vi "InterpretDiagram.vi"(5 "Diagram":refnum<class "Diagram.lvclass">, 6 "error in":errorcluster, 9 "VI Interpreter in":refnum<class "VI Interpreter.lvclass">) -> (0 "error out":errorcluster, 3 "VI Interpreter out":refnum<class "VI Interpreter.lvclass">, 4 "Diagram out":refnum<class "Diagram.lvclass">)   [LabVIEW 2014, in "VI Interpreter.lvclass"]
uses:
  VI Interpreter.lvclass
  Diagram/Diagram.lvclass
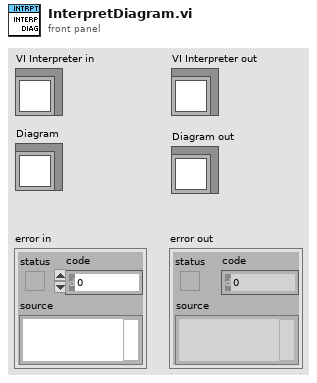
[diagram p1: front panel]
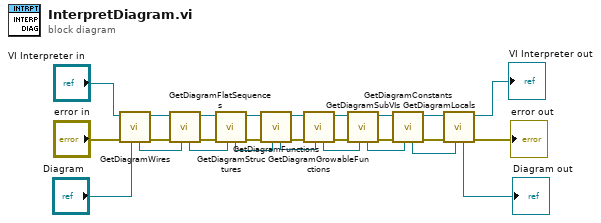
[diagram p0: block diagram]
diagram:
  n1 = call "GetDiagramWires.vi"("Diagram"="Diagram", "error in"="error in", "VI Interpreter in"="VI Interpreter in") -> ("error out"=w6:errorcluster, "VI Interpreter out"=w7:refnum<class "VI Interpreter.lvclass">, "Diagram out"=w5:refnum<class "Diagram.lvclass">)  [unwired: 4 in]
  n2 = call "GetDiagramFlatSequences.vi"("Diagram"=w5, "error in"=w6, "VI Interpreter in"=w7) -> ("error out"=w3:errorcluster, "VI Interpreter out"=w2:refnum<class "VI Interpreter.lvclass">, "Diagram out"=w4:refnum<class "Diagram.lvclass">)  [unwired: 4 in]
  n3 = call "GetDiagramStructures.vi"("Diagram"=w4, "error in"=w3, "VI Interpreter in"=w2) -> ("error out"=w26:errorcluster, "VI Interpreter out"=w27:refnum<class "VI Interpreter.lvclass">, "Diagram out"=w25:refnum<class "Diagram.lvclass">)  [unwired: 4 in]
  n4 = call "GetDiagramFunctions.vi"("Diagram"=w25, "error in"=w26, "VI Interpreter in"=w27) -> ("error out"=w20:errorcluster, "VI Interpreter out"=w24:refnum<class "VI Interpreter.lvclass">, "Diagram out"=w23:refnum<class "Diagram.lvclass">)  [unwired: 4 in]
  n5 = call "GetDiagramGrowableFunctions.vi"("Diagram"=w23, "error in"=w20, "VI Interpreter in"=w24) -> ("error out"=w17:errorcluster, "VI Interpreter out"=w19:refnum<class "VI Interpreter.lvclass">, "Diagram out"=w15:refnum<class "Diagram.lvclass">)  [unwired: 4 in]
  n6 = call "GetDiagramSubVIs.vi"("Diagram"=w15, "error in"=w17, "VI Interpreter in"=w19) -> ("error out"=w16:errorcluster, "VI Interpreter out"=w18:refnum<class "VI Interpreter.lvclass">, "Diagram out"=w14:refnum<class "Diagram.lvclass">)  [unwired: 4 in]
  n7 = call "GetDiagramConstants.vi"("Diagram"=w14, "error in"=w16, "VI Interpreter in"=w18) -> ("error out"=w12:errorcluster, "VI Interpreter out"=w13:refnum<class "VI Interpreter.lvclass">, "Diagram out"=w11:refnum<class "Diagram.lvclass">)  [unwired: 4 in]
  n8 = call "GetDiagramLocals.vi"("Diagram"=w11, "error in"=w12, "VI Interpreter in"=w13) -> ("error out"=→"error out":errorcluster, "VI Interpreter out"=→"VI Interpreter out":refnum<class "VI Interpreter.lvclass">, "Diagram out"=→"Diagram out":refnum<class "Diagram.lvclass">)  [unwired: 4 in]
